vi "calculate_total_length.vi"(8 "error in (no error)":errorcluster, 11 "TrajectoryDL091126GenericVoxel in":refnum<class "TrajectoryDL091126GenericVoxel.lvclass">) -> (0 "error out":errorcluster, 1 "inter-pixel distance":dbl[unit], 2 "total length":dbl[unit], 3 "TrajectoryDL091126GenericVoxel out":refnum<class "TrajectoryDL091126GenericVoxel.lvclass">)   [LabVIEW 2010, in "TrajectoryDL091126GenericVoxel.lvclass"]
uses:
  TrajectoryDL091126GenericVoxel.lvclass
  common/classes/ErrorController/ErrorController/class_data.vi
  common/classes/SpaceVector/SpaceVector/SpaceVector.lvclass
  common/classes/ErrorController/ErrorController/ErrorController.lvclass
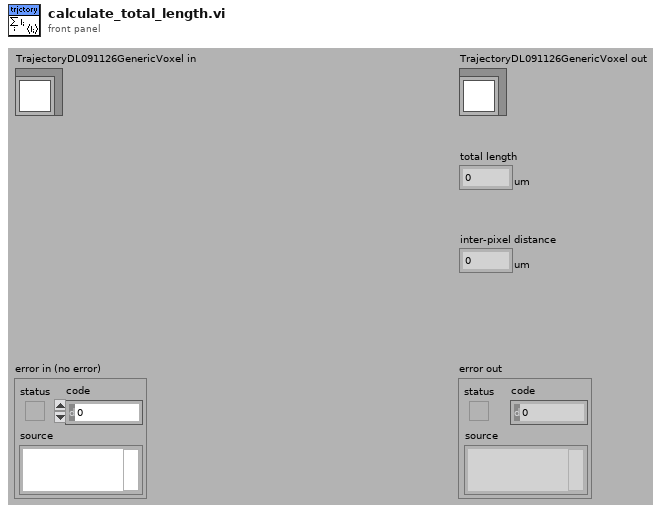
[diagram p1: front panel]
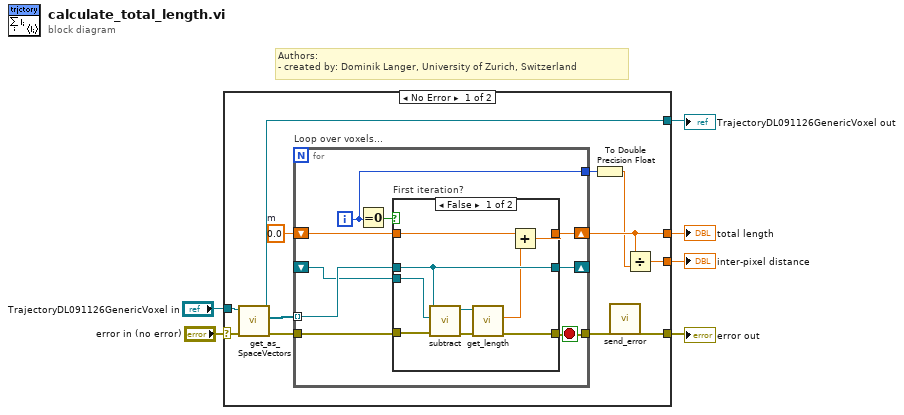
[diagram p0: block diagram]
diagram:
  # "Authors: \n- created by: Dominik Langer, University of Zurich, Switzerland"
  n1 = case shown="No Error" "error in (no error)" {
    selector: "error in (no error)" -> [w13 w41]
    tunnel: [w8 w41] -> w5
    tunnel: [w9 w40] -> w3
    tunnel: "TrajectoryDL091126GenericVoxel in" -> [w12 w40]
    tunnel: [w16 _] -> w2
    tunnel: [w14 _] -> w1
    frame No Error {
      w18 = dbl[unit] 0.0  # m
      n2 = call-dynamic "get_as_SpaceVectors.vi"("error in (no error)"=w13, "TrajectoryDL091126GenericVoxel in"=w12) -> ("error out"=w11:errorcluster, "voxels"=w10:refnum<class "SpaceVector.lvclass">[], "TrajectoryDL091126GenericVoxel out"=w9:refnum<class "TrajectoryDL091126GenericVoxel.lvclass">)  [unwired: 6 in, 1 out]
      n3 = for "Loop over voxels..." {
        shift-right: [w27] -> w16
        shift-left: w18 -> [w26]
        tunnel: [w21] -> w17
        tunnel: w10 -> [w24] mode=indexing
        shift-right: [w23] -> _
        shift-left: _ -> [w22]
        tunnel: w11 -> [w25]
        tunnel: [w19] -> w7
        i -> [w21]
        stop <- w19 stop-if-true
        n4 = Equal To 0?(x=w21) -> (x = 0?=w20:bool)
        n5 = case "First iteration?" shown="False" w20 {
          tunnel: [w35 w39] -> w27
          tunnel: w26 -> [w36 w39]
          tunnel: w25 -> [w34 w38]
          tunnel: w24 -> [w33 w37]
          tunnel: [w33 w37] -> w23
          tunnel: w22 -> [w32 _]
          tunnel: [w29 w38] -> w19
          frame False {
            n6 = call "subtract.vi"("error in (no error)"=w34, "subtrahend"=w32, "SpaceVector in"=w33) -> ("error out"=w31:errorcluster, "SpaceVector out"=w30:refnum<class "SpaceVector.lvclass">)  [unwired: 7 in]
            n7 = call "get_length.vi"("error in (no error)"=w31, "SpaceVector in"=w30) -> ("error out"=w29:errorcluster, "length"=w28:dbl[unit])  [unwired: 7 in, 1 out]
            n8 = Add(x=w36, y=w28) -> (x+y=w35:dbl[unit])
          }
          frame True {
            # "Skip first iteration..."
          }
        }
      }
      n9 = To Double Precision Float(number=w17) -> (double precision float=w15:dbl)
      n10 = call "send_error.vi"("error in (no error)"=w7) -> ("error out"=w8:errorcluster)  [unwired: 10 in]
      n11 = Divide(x=w16, y=w15) -> (x/y=w14:dbl[unit])
    }
    frame Error {
    }
  }
  "error out" <- w5
  "TrajectoryDL091126GenericVoxel out" <- w3
  "total length" <- w2
  "inter-pixel distance" <- w1
